vi "bandejasXML_to_ArrayClusters.vi"(0 "path":path, 5 "Array Clusters Bandejas":T1, 7 "Filenames":string[](array[string]), 9 "Nombres bandejas":string[](array[string]), 11 "error in (no error)":errorcluster) -> (3 "Nombres bandejas":string[](array[string]), 4 "filenames":string[](array[string]), 10 "Array Clusters Bandejas":T1, 15 "error out":errorcluster)   [LabVIEW 2019]
uses:
  Type_defs/Array_deClusterBandeja.ctl
  Type_defs/Data_Bandeja.ctl
  <vilib>/Utility/xml.llb/Read From XML File(array).vi
  <vilib>/Utility/error.llb/Error Cluster From Error Code.vi
  <vilib>/ErrorRing/Error Ring.xnode
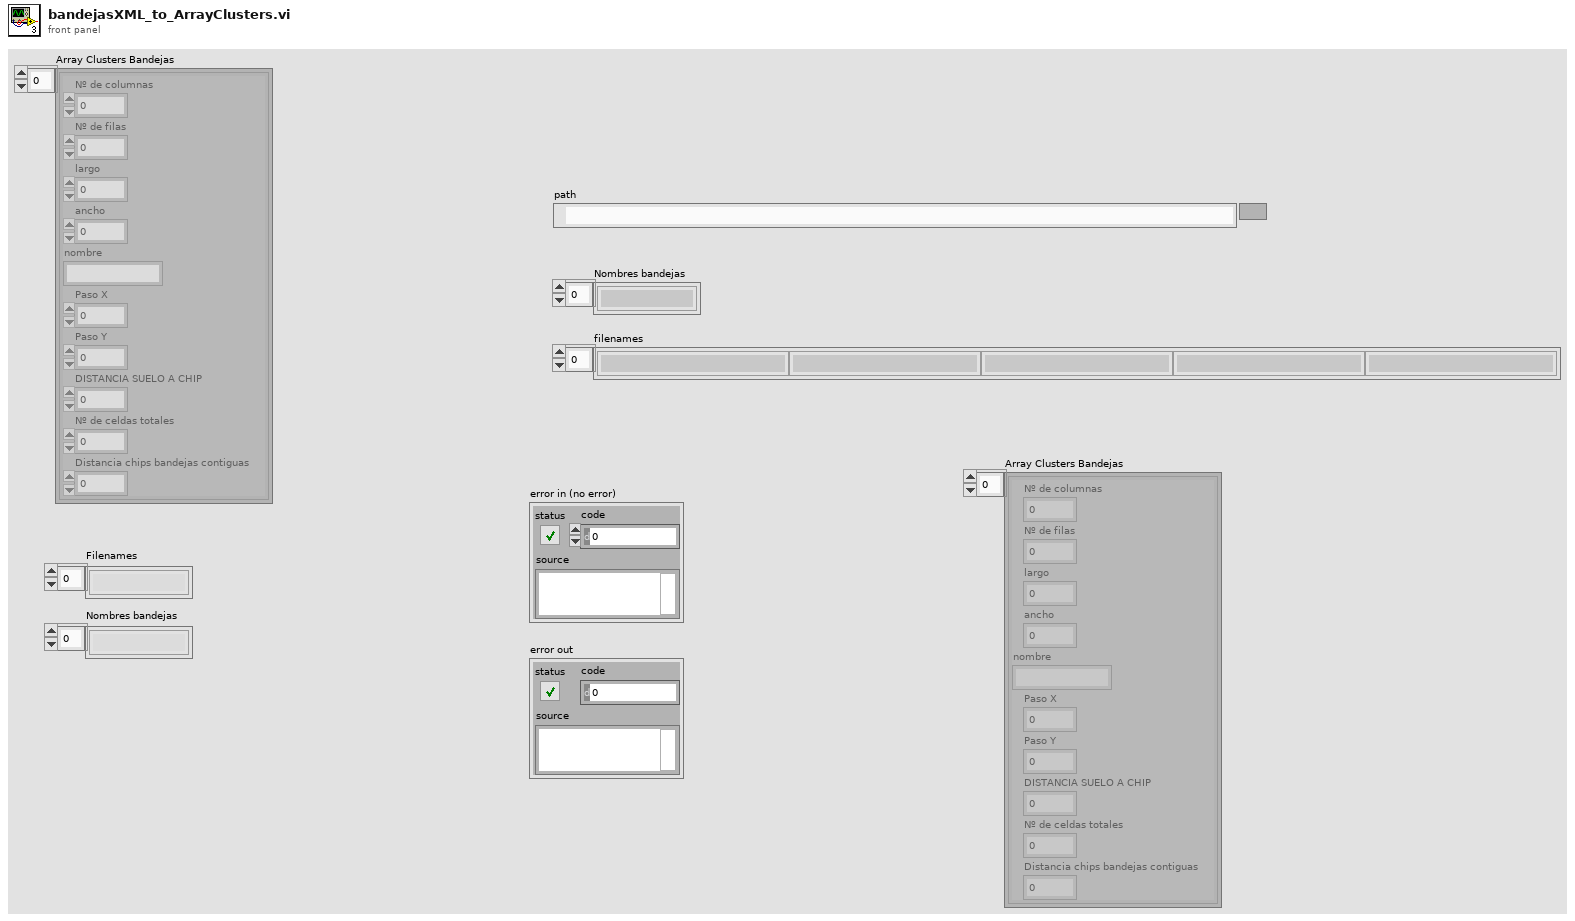
[diagram p1: front panel]
types:
  T1 = typedef "Array_deClusterBandeja.ctl" = cluster{"Nº de columnas ":u32, "Nº de filas ":u32, "largo":u32, "ancho":u32, "nombre":string, "Paso X":dbl, "Paso Y":dbl, "DISTANCIA SUELO A CHIP  ":dbl, "Nº de celdas totales":u16, "Distancia chips bandejas contiguas":dbl}[]
  T2 = typedef "Data_Bandeja.ctl" = cluster{"Nº de columnas ":u32, "Nº de filas ":u32, "largo":u32, "ancho":u32, "nombre":string, "Paso X (en mm)":dbl, "Paso Y (en mm)":dbl, "DISTANCIA SUELO A CHIP  ":dbl, "Nº de celdas totales":u16, "Distancia chips bandejas contiguas":dbl}
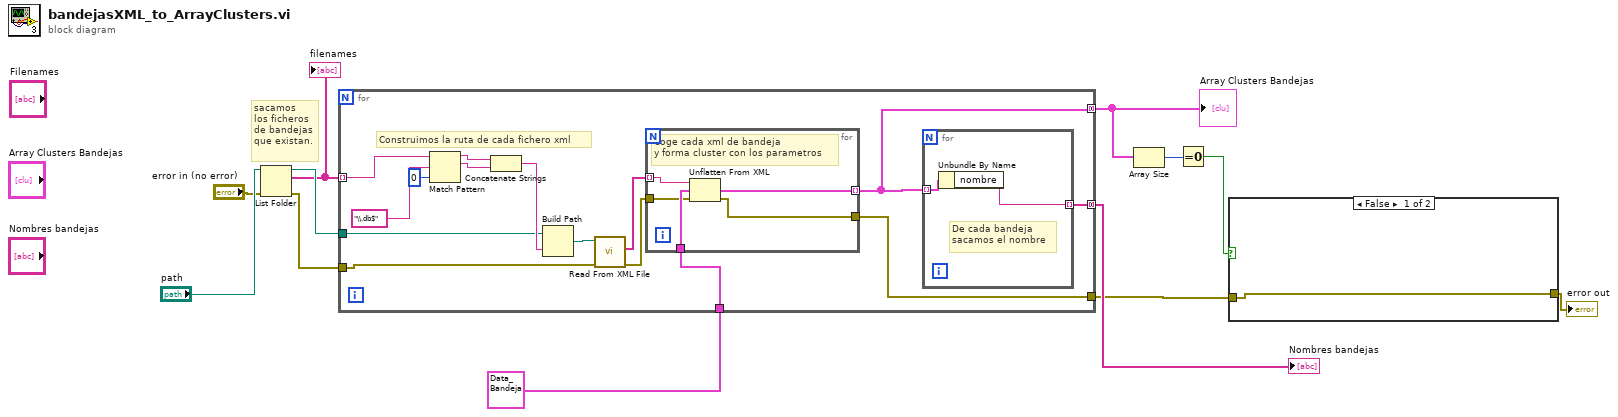
[diagram p0: block diagram]
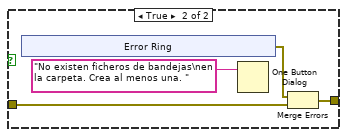
[diagram p2: hidden frame]
diagram:
  # "sacamos\nlos ficheros\nde bandejas\nque existan."
  n1 = List Folder(path="path", error in="error in (no error)") -> (path out=w12:path, filenames=w7:string[], error out=w8:errorcluster)  [unwired: 2 in, 1 out]
  "filenames" <- w7
  n2 = for {
    tunnel: w7 -> [w27] mode=indexing
    tunnel: w12 -> [w21]
    tunnel: w8 -> [w18]
    tunnel: T2 {"Nº de columnas "=0, "Nº de filas "=0, "largo"=0, "ancho"=0, "nombre"="nombre", "Paso X (en mm)"=0.0, "Paso Y (en mm)"=0.0, "DISTANCIA SUELO A CHIP  "=0.0, "Nº de celdas totales"=0, "Distancia chips bandejas contiguas"=0.0} -> [w17]
    tunnel: [w16] -> w11 mode=concatenating
    tunnel: [w15] -> w1 mode=concatenating
    tunnel: [w13] -> w6
    # "Construimos la ruta de cada fichero xml"
    n3 = Match Pattern(string=w27, regular expression="\\.db$", offset (0)=0) -> (before substring=w24:string, match substring=w23:string)  [unwired: 2 out]
    n4 = Concatenate Strings(w24, w23) -> (w22:string)
    n5 = Build Path(base path=w21, name or relative path=w22) -> (appended path=w19:path)
    n6 = call-poly <vilib>:"Read From XML File.vi"("error in (no error)"=w18, "XML File Path"=w19) -> ("error out"=w14:errorcluster, "XML Elements"=w20:string[])  [unwired: 7 in, 1 out]
    n7 = for {
      tunnel: w20 -> [w34] mode=indexing
      tunnel: [w33] -> w15 mode=indexing
      tunnel: w17 -> [w32]
      tunnel: w14 -> [w31]
      tunnel: [w30] -> w13
      # "Coge cada xml de bandeja\ny forma cluster con los parametros"
      n8 = Unflatten From XML(xml string=w34, type=w32, error in (no error)=w31) -> (value=w33:T2, error out=w30:errorcluster)
    }
    n9 = for {
      tunnel: [w29] -> w16 mode=indexing
      tunnel: w15 -> [w28] mode=indexing
      # "De cada bandeja\nsacamos el nombre"
      n10 = Unbundle By Name(w28) -> ("nombre"=w29:string)
    }
  }
  "Nombres bandejas" <- w11
  "Array Clusters Bandejas" <- w1
  n11 = Array Size(array=w1) -> (size(s)=w5:i32)
  n12 = Equal To 0?(x=w5) -> (x = 0?=w4:bool)
  n13 = case shown="False" w4 {
    tunnel: w6 -> [w35 w39]
    tunnel: [w35 w37] -> w3
    frame False {
    }
    frame True {
      n14 = xnode "Error Ring"() -> ("error out"=w38:errorcluster)
      n15 = One Button Dialog(message="No existen ficheros de bandejas\nen la carpeta. Crea al menos una. ") -> ()  [unwired: 1 in, 1 out]
      n16 = Merge Errors(w38, w39) -> (w37:errorcluster)
    }
  }
  "error out" <- w3
